vi "read_Mazak.vi"(8 "error in":errorcluster, 10 "Boolean":bool=TRUE, 11 "URL":string) -> (0 "machine":T2, 1 "c2":T4, 2 "c":T5, 3 "vr":T3, 4 "position":T1, 5 "br":T6, 7 "error out":errorcluster)   [LabVIEW 2014]
uses:
  <vilib>/addons/internet/NI_InternetTK_Core_VIs.lvlib
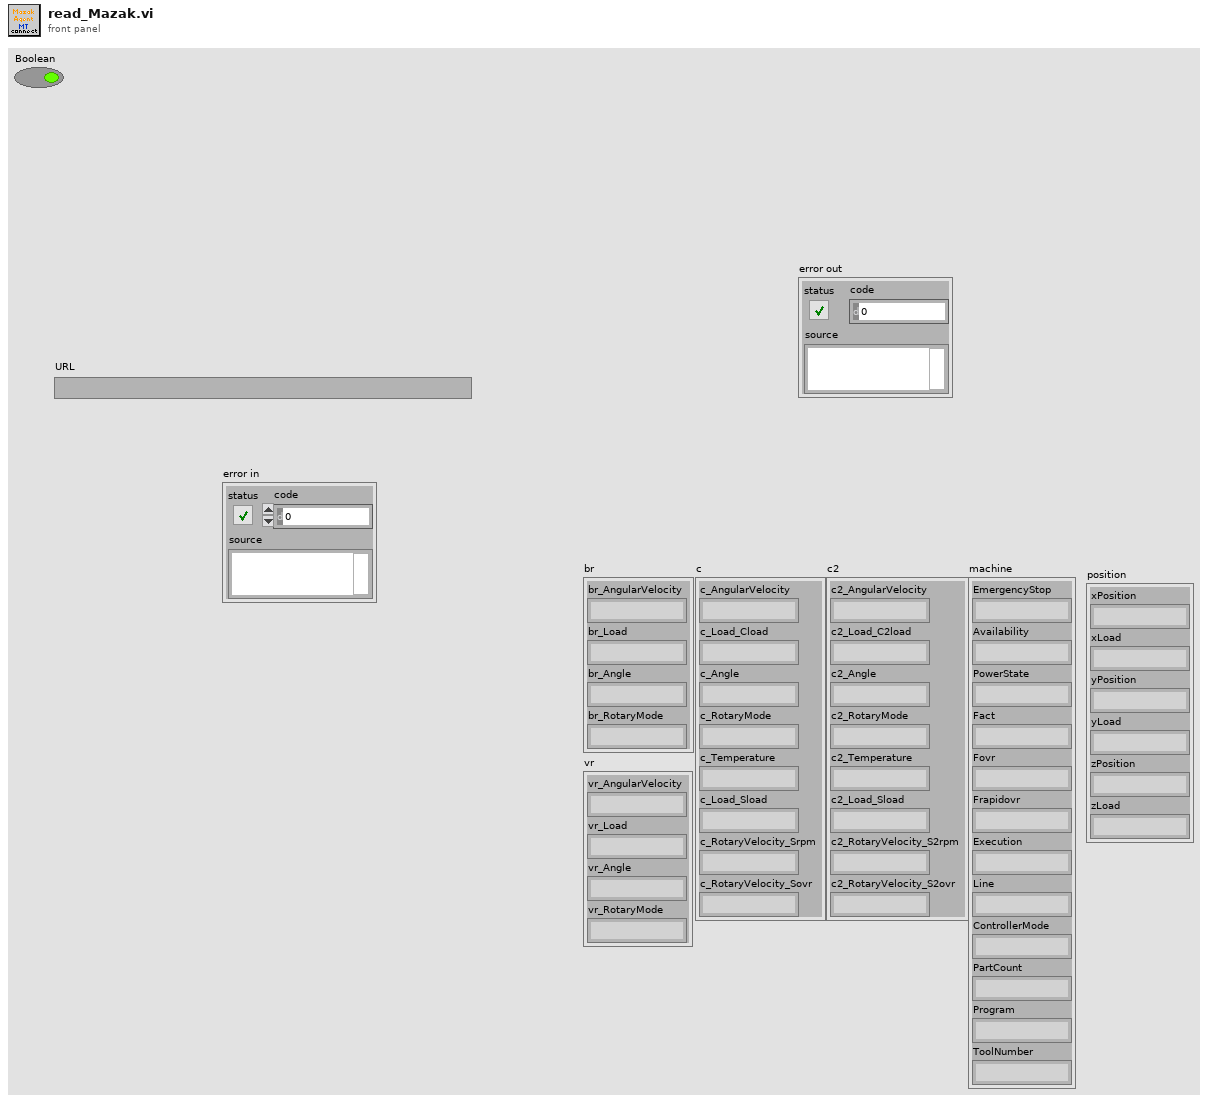
[diagram p1: front panel]
types:
  T1 = cluster{"xPosition":string, "xLoad":string, "yPosition":string, "yLoad":string, "zPosition":string, "zLoad":string}
  T2 = cluster{"EmergencyStop":string, "Availability":string, "PowerState":string, "Fact":string, "Fovr":string, "Frapidovr":string, "Execution":string, "Line":string, "ControllerMode":string, "PartCount":string, "Program":string, "ToolNumber":string}
  T3 = cluster{"vr_AngularVelocity":string, "vr_Load":string, "vr_Angle":string, "vr_RotaryMode":string}
  T4 = cluster{"c2_AngularVelocity":string, "c2_Load_C2load":string, "c2_Angle":string, "c2_RotaryMode":string, "c2_Temperature":string, "c2_Load_Sload":string, "c2_RotaryVelocity_S2rpm":string, "c2_RotaryVelocity_S2ovr":string}
  T5 = cluster{"c_AngularVelocity":string, "c_Load_Cload":string, "c_Angle":string, "c_RotaryMode":string, "c_Temperature":string, "c_Load_Sload":string, "c_RotaryVelocity_Srpm":string, "c_RotaryVelocity_Sovr":string}
  T6 = cluster{"br_AngularVelocity":string, "br_Load":string, "br_Angle":string, "br_RotaryMode":string}
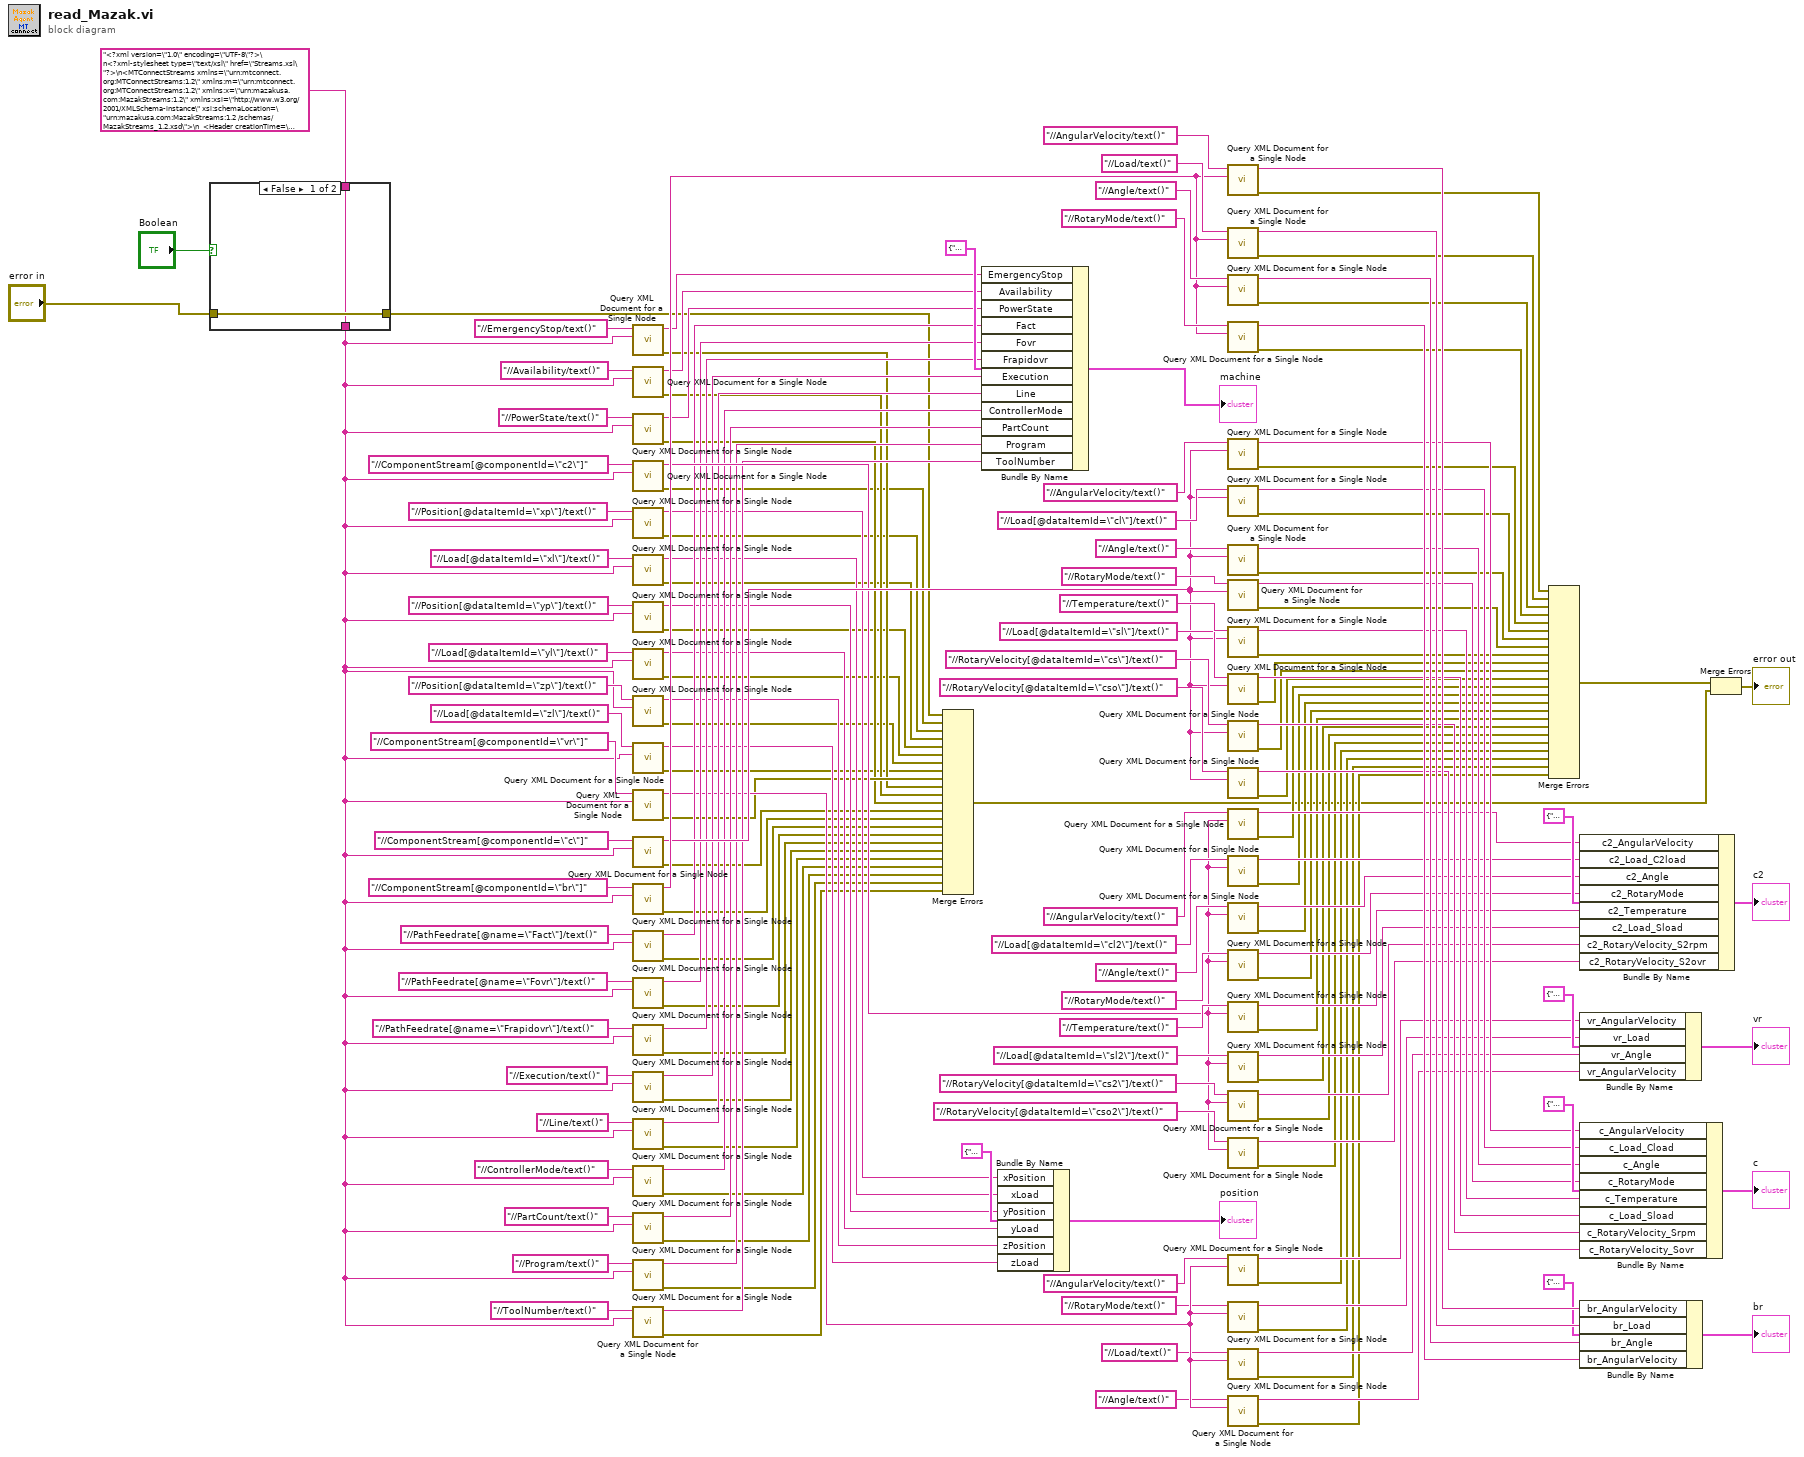
[diagram p0: block diagram]
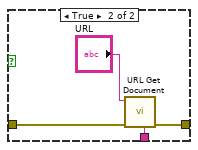
[diagram p2: hidden frame]
diagram:
  n1 = case shown="False" "Boolean" {
    tunnel: "error in" -> [w160 w164]
    tunnel: [w159 w163] -> w53
    tunnel: [w160 w161] -> w3
    tunnel: "<?xml version=\"1.0\" encoding=\"UTF-8\"?>\n<?xml-stylesheet type=\"text/xsl\" href=\"Streams.xsl\"?>\n<MTConnectStreams xmlns=\"urn:mtconnect.org:MTConnectStreams:1.2\" xmlns:m=\"urn:mtconnect.org:MTConnectStreams:1.2\" xmlns:x=\"urn:mazakusa.com:MazakStreams:1.2\" xmlns:xsi=\"http://www.w3.org/2001/XMLSchema-instance\" xsi:schemaLocation=\"urn:mazakusa.com:MazakStreams:1.2 /schemas/MazakStreams_1.2.xsd\">\n  <Header creationTime=\"2016-04-06T16:39:26Z\" sender=\"MAZATROL-PC\" instanceId=\"1459800093\" version=\"1.2.0.22\" bufferSize=\"16384\" nextSequence=\"535780\" firstSequence=\"519396\" lastSequence=\"535779\" />\n  <Streams>\n    <DeviceStream name=\"e-Series\" uuid=\"MAZAK-M7303290458\">\n      <ComponentStream component=\"Axes\" name=\"base\" componentId=\"a\">\n        <Condition>\n          <Normal dataItemId=\"servo\" timestamp=\"2016-04-04T20:01:46.125Z\" name=\"servo_cond\" sequence=\"82\" type=\"ACTUATOR\" />\n        </Condition>\n      </ComponentStream>\n      <ComponentStream component=\"Rotary\" name=\"B\" componentId=\"br\">\n        <Samples>\n          <AngularVelocity dataItemId=\"bf\" timestamp=\"2016-04-06T11:27:44.709Z\" name=\"Bfrt\" sequence=\"516876\">0</AngularVelocity>\n          <Load dataItemId=\"bl\" timestamp=\"2016-04-06T11:27:44.709Z\" name=\"Bload\" sequence=\"516877\">0</Load>\n          <Angle dataItemId=\"bpos\" timestamp=\"2016-04-06T11:27:44.709Z\" name=\"Bdeg\" sequence=\"516875\" subType=\"ACTUAL\">0</Angle>\n        </Samples>\n        <Events>\n          <RotaryMode dataItemId=\"brf\" timestamp=\"2016-04-04T20:01:33.224Z\" name=\"brfunc\" sequence=\"6\">UNAVAILABLE</RotaryMode>\n        </Events>\n        <Condition>\n          <Normal dataItemId=\"bt\" timestamp=\"2016-04-04T20:03:10.465Z\" name=\"Btravel\" sequence=\"97\" type=\"ANGLE\" />\n        </Condition>\n      </ComponentStream>\n      <ComponentStream component=\"Rotary\" name=\"C\" componentId=\"c\">\n        <Samples>\n          <AngularVelocity dataItemId=\"cf\" timestamp=\"2016-04-06T11:58:20.995Z\" name=\"Cfrt\" sequence=\"521223\">0</AngularVelocity>\n          <Load dataItemId=\"cl\" timestamp=\"2016-04-06T11:58:20.995Z\" name=\"Cload\" sequence=\"521224\">0</Load>\n          <Angle dataItemId=\"cpos\" timestamp=\"2016-04-06T11:58:20.995Z\" name=\"Cdeg\" sequence=\"521222\" subType=\"ACTUAL\">138.3637</Angle>\n          <RotaryVelocity dataItemId=\"cs\" timestamp=\"2016-04-06T11:39:30.023Z\" name=\"Srpm\" sequence=\"520012\" subType=\"ACTUAL\">0</RotaryVelocity>\n          <RotaryVelocity dataItemId=\"cso\" timestamp=\"2016-04-06T11:03:57.000Z\" name=\"Sovr\" sequence=\"509281\" subType=\"OVERRIDE\">100</RotaryVelocity>\n          <Temperature dataItemId=\"ctemp\" timestamp=\"2016-04-06T16:19:20.460Z\" name=\"Stemp\" sequence=\"534875\">23</Temperature>\n          <Load dataItemId=\"sl\" timestamp=\"2016-04-06T11:24:51.813Z\" name=\"Sload\" sequence=\"516066\">0</Load>\n        </Samples>\n        <Events>\n          <RotaryMode dataItemId=\"rf\" timestamp=\"2016-04-04T20:01:33.224Z\" name=\"crfunc\" sequence=\"46\">UNAVAILABLE</RotaryMode>\n        </Events>\n        <Condition>\n          <Normal dataItemId=\"ct\" timestamp=\"2016-04-04T20:03:10.465Z\" name=\"Ctravel\" sequence=\"98\" type=\"ANGLE\" />\n          <Normal dataItemId=\"spc\" timestamp=\"2016-04-04T20:03:10.465Z\" name=\"Sload_cond\" sequence=\"100\" type=\"LOAD\" />\n          <Normal dataItemId=\"tmp\" timestamp=\"2016-04-04T20:03:10.465Z\" name=\"Stemp_cond\" sequence=\"101\" type=\"TEMPERATURE\" />\n        </Condition>\n      </ComponentStream>\n      <ComponentStream component=\"Rotary\" name=\"C2\" componentId=\"c2\">\n        <Samples>\n          <AngularVelocity dataItemId=\"cf2\" timestamp=\"2016-04-04T20:01:33.224Z\" name=\"C2frt\" sequence=\"10\">UNAVAILABLE</AngularVelocity>\n          <Load dataItemId=\"cl2\" timestamp=\"2016-04-04T20:01:33.224Z\" name=\"C2load\" sequence=\"12\">UNAVAILABLE</Load>\n          <Angle dataItemId=\"cpos2\" timestamp=\"2016-04-04T20:01:33.224Z\" name=\"C2deg\" sequence=\"17\" subType=\"ACTUAL\">UNAVAILABLE</Angle>\n          <RotaryVelocity dataItemId=\"cs2\" timestamp=\"2016-04-04T20:01:33.224Z\" name=\"S2rpm\" sequence=\"19\" subType=\"ACTUAL\">UNAVAILABLE</RotaryVelocity>\n          <RotaryVelocity dataItemId=\"cso2\" timestamp=\"2016-04-04T20:01:33.224Z\" name=\"S2ovr\" sequence=\"21\" subType=\"OVERRIDE\">UNAVAILABLE</RotaryVelocity>\n          <Temperature dataItemId=\"ctemp2\" timestamp=\"2016-04-04T20:01:33.224Z\" name=\"S2temp\" sequence=\"25\">UNAVAILABLE</Temperature>\n          <Load dataItemId=\"sl2\" timestamp=\"2016-04-04T20:01:33.224Z\" name=\"S2load\" sequence=\"51\">UNAVAILABLE</Load>\n        </Samples>\n        <Events>\n          <RotaryMode dataItemId=\"rf2\" timestamp=\"2016-04-04T20:01:33.224Z\" name=\"c2rfunc\" sequence=\"47\">UNAVAILABLE</RotaryMode>\n        </Events>\n        <Condition>\n          <Unavailable dataItemId=\"ct2\" timestamp=\"2016-04-04T20:01:33.224Z\" name=\"C2travel\" sequence=\"23\" type=\"ANGLE\" />\n          <Unavailable dataItemId=\"spc2\" timestamp=\"2016-04-04T20:01:33.224Z\" name=\"S2load_cond\" sequence=\"53\" type=\"LOAD\" />\n          <Unavailable dataItemId=\"tmp2\" timestamp=\"2016-04-04T20:01:33.224Z\" name=\"S2temp_cond\" sequence=\"60\" type=\"TEMPERATURE\" />\n        </Condition>\n      </ComponentStream>\n      <ComponentStream component=\"Controller\" name=\"controller\" componentId=\"cont\">\n        <Events>\n          <EmergencyStop dataItemId=\"estop\" timestamp=\"2016-04-05T13:35:23.466Z\" name=\"estop\" sequence=\"199888\">ARMED</EmergencyStop>\n        </Events>\n        <Condition>\n          <Normal dataItemId=\"ccond\" timestamp=\"2016-04-04T20:01:46.125Z\" name=\"comms_cond\" sequence=\"83\" type=\"COMMUNICATIONS\" />\n          <Normal dataItemId=\"logic\" timestamp=\"2016-04-06T16:39:04.533Z\" name=\"logic_cond\" sequence=\"535758\" type=\"LOGIC_PROGRAM\" />\n          <Normal dataItemId=\"system\" timestamp=\"2016-04-06T11:27:43.618Z\" name=\"system_cond\" sequence=\"516862\" type=\"SYSTEM\" />\n        </Condition>\n      </ComponentStream>\n      <ComponentStream component=\"Coolant\" name=\"coolant\" componentId=\"coolant\">\n        <Condition>\n          <Normal dataItemId=\"coollevel\" timestamp=\"2016-04-06T08:34:22.682Z\" name=\"coolant_level\" sequence=\"435644\" type=\"LEVEL\" />\n          <Normal dataItemId=\"coolpress\" timestamp=\"2016-04-04T20:01:46.125Z\" name=\"coolant_pres\" sequence=\"90\" type=\"PRESSURE\" />\n          <Normal dataItemId=\"cooltemp\" timestamp=\"2016-04-04T20:01:46.125Z\" name=\"coolant_temp\" sequence=\"89\" type=\"TEMPERATURE\" />\n        </Condition>\n      </ComponentStream>\n      <ComponentStream component=\"Device\" name=\"e-Series\" componentId=\"d1\">\n        <Events>\n          <Availability dataItemId=\"avail\" timestamp=\"2016-04-04T20:01:46.125Z\" sequence=\"81\">AVAILABLE</Availability>\n          <AssetChanged dataItemId=\"d1_asset_chg\" timestamp=\"2016-04-04T20:01:33.224Z\" sequence=\"27\" assetType=\"\">UNAVAILABLE</AssetChanged>\n        </Events>\n      </ComponentStream>\n      <ComponentStream component=\"Electric\" name=\"electric\" componentId=\"elec\">\n        <Events>\n          <PowerState dataItemId=\"pwr\" timestamp=\"2016-04-04T20:03:10.465Z\" name=\"power\" sequence=\"93\">ON</PowerState>\n        </Events>\n        <Condition>\n          <Normal dataItemId=\"pwrt\" timestamp=\"2016-04-04T20:01:46.125Z\" name=\"electric_temp\" sequence=\"92\" type=\"TEMPERATURE\" />\n        </Condition>\n      </ComponentStream>\n      <ComponentStream component=\"Hydraulic\" name=\"hydraulic\" componentId=\"hydraulic\">\n        <Condition>\n          <Normal dataItemId=\"hyd\" timestamp=\"2016-04-04T20:01:46.125Z\" name=\"hydra_cond\" sequence=\"87\" type=\"PRESSURE\" />\n        </Condition>\n      </ComponentStream>\n      <ComponentStream component=\"Path\" name=\"path\" componentId=\"path1\">\n        <Samples>\n          <AccumulatedTime dataItemId=\"atime\" timestamp=\"2016-04-06T11:39:37.593Z\" name=\"auto_time\" sequence=\"520070\" subType=\"x:AUTO\">32773294</AccumulatedTime>\n          <AccumulatedTime dataItemId=\"ctime\" timestamp=\"2016-04-06T11:39:28.947Z\" name=\"cut_time\" sequence=\"520008\" subType=\"x:CUT\">14501503</AccumulatedTime>\n          <PathFeedrate dataItemId=\"pf\" timestamp=\"2016-04-06T11:58:20.995Z\" name=\"Fact\" sequence=\"521225\" subType=\"ACTUAL\">0</PathFeedrate>\n          <PathFeedrate dataItemId=\"pfo\" timestamp=\"2016-04-06T11:24:53.997Z\" name=\"Fovr\" sequence=\"516086\" subType=\"OVERRIDE\">100</PathFeedrate>\n          <PathFeedrate dataItemId=\"pfr\" timestamp=\"2016-04-06T11:39:40.145Z\" name=\"Frapidovr\" sequence=\"520075\" subType=\"OVERRIDE\">100</PathFeedrate>\n          <AccumulatedTime dataItemId=\"yltime\" timestamp=\"2016-04-06T16:39:26.264Z\" name=\"total_time\" sequence=\"535779\" subType=\"x:TOTAL\">71278506</AccumulatedTime>\n        </Samples>\n        <Events>\n          <Execution dataItemId=\"exec\" timestamp=\"2016-04-06T11:39:40.145Z\" name=\"execution\" sequence=\"520074\">STOPPED</Execution>\n          <Line dataItemId=\"ln\" timestamp=\"2016-04-06T11:39:37.593Z\" name=\"line\" sequence=\"520067\">0</Line>\n          <ControllerMode dataItemId=\"mode\" timestamp=\"2016-04-06T11:39:40.145Z\" name=\"mode\" sequence=\"520076\">MANUAL</ControllerMode>\n          <PartCount dataItemId=\"pc\" timestamp=\"2016-04-04T20:03:11.916Z\" name=\"PartCountAct\" sequence=\"139\">0</PartCount>\n          <x:ProgramComment dataItemId=\"pcmt\" timestamp=\"2016-04-05T19:02:24.670Z\" name=\"program_cmt\" sequence=\"265033\" />\n          <Program dataItemId=\"pgm\" timestamp=\"2016-04-06T08:34:29.153Z\" name=\"program\" sequence=\"435652\">555885</Program>\n          <x:PalletNum dataItemId=\"pltnum\" timestamp=\"2016-04-04T20:03:13.211Z\" name=\"pallet_num\" sequence=\"143\">2</x:PalletNum>\n          <x:SequenceNumber dataItemId=\"seq\" timestamp=\"2016-04-06T11:39:37.593Z\" name=\"sequenceNum\" sequence=\"520069\">0</x:SequenceNumber>\n          <x:ProgramComment dataItemId=\"spcmt\" timestamp=\"2016-04-06T08:28:01.332Z\" name=\"subprogram_cmt\" sequence=\"434132\" subType=\"x:SUB\" />\n          <Program dataItemId=\"spgm\" timestamp=\"2016-04-06T11:27:35.278Z\" name=\"subprogram\" sequence=\"516799\" subType=\"x:SUB\" />\n          <ToolNumber dataItemId=\"tid\" timestamp=\"2016-04-06T11:27:29.889Z\" name=\"Tool_number\" sequence=\"516764\">16</ToolNumber>\n          <x:ToolGroup dataItemId=\"tid1\" timestamp=\"2016-04-04T20:03:11.916Z\" name=\"Tool_group\" sequence=\"136\">0</x:ToolGroup>\n          <x:ToolSuffix dataItemId=\"tsuf1\" timestamp=\"2016-04-04T20:01:33.224Z\" name=\"Tool_suffix\" sequence=\"61\">UNAVAILABLE</x:ToolSuffix>\n          <x:Unit dataItemId=\"unit\" timestamp=\"2016-04-04T20:03:11.916Z\" name=\"unitNum\" sequence=\"138\">0</x:Unit>\n        </Events>\n        <Condition>\n          <Normal dataItemId=\"motion\" timestamp=\"2016-04-05T15:21:48.586Z\" name=\"motion_cond\" sequence=\"233870\" type=\"MOTION_PROGRAM\" />\n          <Normal dataItemId=\"path_system\" timestamp=\"2016-04-04T20:03:10.465Z\" name=\"path_system\" sequence=\"103\" type=\"SYSTEM\" />\n        </Condition>\n      </ComponentStream>\n      <ComponentStream component=\"Pneumatic\" name=\"pneumatic\" componentId=\"pneumatic\">\n        <Condition>\n          <Normal dataItemId=\"pneupress\" timestamp=\"2016-04-05T08:03:22.286Z\" name=\"pneu_cond\" sequence=\"131871\" type=\"PRESSURE\" />\n        </Condition>\n      </ComponentStream>\n      <ComponentStream component=\"Rotary\" name=\"V\" componentId=\"vr\">\n        <Samples>\n          <AngularVelocity dataItemId=\"vf\" timestamp=\"2016-04-04T20:03:11.916Z\" name=\"Vfrt\" sequence=\"122\">0</AngularVelocity>\n          <Load dataItemId=\"vl\" timestamp=\"2016-04-04T20:03:11.916Z\" name=\"Vload\" sequence=\"123\">0</Load>\n          <Angle dataItemId=\"vpos\" timestamp=\"2016-04-04T20:03:11.916Z\" name=\"Vdeg\" sequence=\"121\" subType=\"ACTUAL\">0</Angle>\n        </Samples>\n        <Events>\n          <RotaryMode dataItemId=\"vrf\" timestamp=\"2016-04-04T20:01:33.224Z\" name=\"vrfunc\" sequence=\"66\">UNAVAILABLE</RotaryMode>\n        </Events>\n        <Condition>\n          <Normal dataItemId=\"vt\" timestamp=\"2016-04-04T20:03:10.465Z\" name=\"Vtravel\" sequence=\"99\" type=\"ANGLE\" />\n        </Condition>\n      </ComponentStream>\n      <ComponentStream component=\"Linear\" name=\"X\" componentId=\"x\">\n        <Samples>\n          <AxisFeedrate dataItemId=\"xf\" timestamp=\"2016-04-06T11:58:12.291Z\" name=\"Xfrt\" sequence=\"521195\">0</AxisFeedrate>\n          <Load dataItemId=\"xl\" timestamp=\"2016-04-06T15:27:46.990Z\" name=\"Xload\" sequence=\"532523\">2</Load>\n          <Position dataItemId=\"xp\" timestamp=\"2016-04-06T11:58:11.214Z\" name=\"Xabs\" sequence=\"521190\" subType=\"ACTUAL\">1334.898524</Position>\n        </Samples>\n        <Condition>\n          <Normal dataItemId=\"xt\" timestamp=\"2016-04-05T04:05:33.224Z\" name=\"Xtravel\" sequence=\"102549\" type=\"POSITION\" />\n        </Condition>\n      </ComponentStream>\n      <ComponentStream component=\"Linear\" name=\"Y\" componentId=\"y\">\n        <Samples>\n          <AxisFeedrate dataItemId=\"yf\" timestamp=\"2016-04-06T11:39:34.344Z\" name=\"Yfrt\" sequence=\"520050\">0</AxisFeedrate>\n          <Load dataItemId=\"yl\" timestamp=\"2016-04-06T11:39:34.344Z\" name=\"Yload\" sequence=\"520051\">3</Load>\n          <Position dataItemId=\"yp\" timestamp=\"2016-04-06T11:39:34.344Z\" name=\"Yabs\" sequence=\"520049\" subType=\"ACTUAL\">529.98243</Position>\n        </Samples>\n        <Condition>\n          <Normal dataItemId=\"yt\" timestamp=\"2016-04-04T20:03:10.465Z\" name=\"Ytravel\" sequence=\"95\" type=\"POSITION\" />\n        </Condition>\n      </ComponentStream>\n      <ComponentStream component=\"Linear\" name=\"Z\" componentId=\"z\">\n        <Samples>\n          <AxisFeedrate dataItemId=\"zf\" timestamp=\"2016-04-06T11:39:32.176Z\" name=\"Zfrt\" sequence=\"520031\">0</AxisFeedrate>\n          <Load dataItemId=\"zl\" timestamp=\"2016-04-06T11:39:33.268Z\" name=\"Zload\" sequence=\"520044\">42</Load>\n          <Position dataItemId=\"zp\" timestamp=\"2016-04-06T11:39:40.145Z\" name=\"Zabs\" sequence=\"520073\" subType=\"ACTUAL\">936.407957</Position>\n        </Samples>\n        <Condition>\n          <Normal dataItemId=\"zt\" timestamp=\"2016-04-04T20:03:10.465Z\" name=\"Ztravel\" sequence=\"96\" type=\"POSITION\" />\n        </Condition>\n      </ComponentStream>\n    </DeviceStream>\n  </Streams>\n</MTConnectStreams>\n" ("XML Input") -> [w159 _]
    frame False {
    }
    frame True {
      n2 = call <vilib>:"URL Get Document.vi"("error in (no error)"=w164, "URL"="URL") -> ("error out"=w161:errorcluster, "content"=w163:string)  [unwired: 5 in, 3 out]
    }
  }
  n3 = call "Query XML Document for a Single Node.vi"("XML document"=w53, "XPath expression"="//EmergencyStop/text()") -> ("error out"=w27:errorcluster, "Result XML"=w96:string)  [unwired: 7 in, 1 out]
  n4 = call "Query XML Document for a Single Node.vi"("XML document"=w53, "XPath expression"="//Availability/text()") -> ("error out"=w26:errorcluster, "Result XML"=w95:string)  [unwired: 7 in, 1 out]
  n5 = call "Query XML Document for a Single Node.vi"("XML document"=w53, "XPath expression"="//PowerState/text()") -> ("error out"=w25:errorcluster, "Result XML"=w94:string)  [unwired: 7 in, 1 out]
  n6 = call "Query XML Document for a Single Node.vi"("XML document"=w53, "XPath expression"="//ComponentStream[@componentId=\"c2\"]") -> ("error out"=w7:errorcluster, "Result XML"=w134:string)  [unwired: 7 in, 1 out]
  n7 = call "Query XML Document for a Single Node.vi"("XML document"=w53, "XPath expression"="//Position[@dataItemId=\"xp\"]/text()") -> ("error out"=w8:errorcluster, "Result XML"=w66:string)  [unwired: 7 in, 1 out]
  n8 = call "Query XML Document for a Single Node.vi"("XML document"=w53, "XPath expression"="//Load[@dataItemId=\"xl\"]/text()") -> ("error out"=w9:errorcluster, "Result XML"=w65:string)  [unwired: 7 in, 1 out]
  n9 = call "Query XML Document for a Single Node.vi"("XML document"=w53, "XPath expression"="//Position[@dataItemId=\"yp\"]/text()") -> ("error out"=w10:errorcluster, "Result XML"=w64:string)  [unwired: 7 in, 1 out]
  n10 = call "Query XML Document for a Single Node.vi"("XML document"=w53, "XPath expression"="//Load[@dataItemId=\"yl\"]/text()") -> ("error out"=w11:errorcluster, "Result XML"=w63:string)  [unwired: 7 in, 1 out]
  n11 = call "Query XML Document for a Single Node.vi"("XML document"=w53, "XPath expression"="//Position[@dataItemId=\"zp\"]/text()") -> ("error out"=w12:errorcluster, "Result XML"=w62:string)  [unwired: 7 in, 1 out]
  n12 = call "Query XML Document for a Single Node.vi"("XML document"=w53, "XPath expression"="//Load[@dataItemId=\"zl\"]/text()") -> ("error out"=w13:errorcluster, "Result XML"=w61:string)  [unwired: 7 in, 1 out]
  n13 = call "Query XML Document for a Single Node.vi"("XML document"=w53, "XPath expression"="//ComponentStream[@componentId=\"vr\"]") -> ("error out"=w28:errorcluster, "Result XML"=w84:string)  [unwired: 7 in, 1 out]
  n14 = call "Query XML Document for a Single Node.vi"("XML document"=w53, "XPath expression"="//ComponentStream[@componentId=\"c\"]") -> ("error out"=w21:errorcluster, "Result XML"=w143:string)  [unwired: 7 in, 1 out]
  n15 = call "Query XML Document for a Single Node.vi"("XML document"=w53, "XPath expression"="//ComponentStream[@componentId=\"br\"]") -> ("error out"=w20:errorcluster, "Result XML"=w149:string)  [unwired: 7 in, 1 out]
  n16 = call "Query XML Document for a Single Node.vi"("XML document"=w53, "XPath expression"="//PathFeedrate[@name=\"Fact\"]/text()") -> ("error out"=w24:errorcluster, "Result XML"=w93:string)  [unwired: 7 in, 1 out]
  n17 = call "Query XML Document for a Single Node.vi"("XML document"=w53, "XPath expression"="//PathFeedrate[@name=\"Fovr\"]/text()") -> ("error out"=w23:errorcluster, "Result XML"=w92:string)  [unwired: 7 in, 1 out]
  n18 = call "Query XML Document for a Single Node.vi"("XML document"=w53, "XPath expression"="//PathFeedrate[@name=\"Frapidovr\"]/text()") -> ("error out"=w22:errorcluster, "Result XML"=w91:string)  [unwired: 7 in, 1 out]
  n19 = call "Query XML Document for a Single Node.vi"("XML document"=w53, "XPath expression"="//Execution/text()") -> ("error out"=w19:errorcluster, "Result XML"=w90:string)  [unwired: 7 in, 1 out]
  n20 = call "Query XML Document for a Single Node.vi"("XML document"=w53, "XPath expression"="//Line/text()") -> ("error out"=w18:errorcluster, "Result XML"=w89:string)  [unwired: 7 in, 1 out]
  n21 = call "Query XML Document for a Single Node.vi"("XML document"=w53, "XPath expression"="//ControllerMode/text()") -> ("error out"=w17:errorcluster, "Result XML"=w88:string)  [unwired: 7 in, 1 out]
  n22 = call "Query XML Document for a Single Node.vi"("XML document"=w53, "XPath expression"="//PartCount/text()") -> ("error out"=w16:errorcluster, "Result XML"=w87:string)  [unwired: 7 in, 1 out]
  n23 = call "Query XML Document for a Single Node.vi"("XML document"=w53, "XPath expression"="//Program/text()") -> ("error out"=w15:errorcluster, "Result XML"=w86:string)  [unwired: 7 in, 1 out]
  n24 = call "Query XML Document for a Single Node.vi"("XML document"=w53, "XPath expression"="//ToolNumber/text()") -> ("error out"=w14:errorcluster, "Result XML"=w85:string)  [unwired: 7 in, 1 out]
  n25 = Merge Errors(w3, w7, w8, w9, w10, w11, w12, w13, w28, w27, w26, w25, w21, w20, w24, w23, w22, w19, w18, w17, w16, w15, w14) -> (w5:errorcluster)
  n26 = Bundle By Name(cluster=T2 {"EmergencyStop"="ARMED", "Availability"="AVAILABLE", "PowerState"="ON", "Fact"="0", "Fovr"="100", "Frapidovr"="100", "Execution"="STOPPED", "Line"="0", "ControllerMode"="MANUAL", "PartCount"="0", "Program"="0", "ToolNumber"="0"} ("input cluster"), "EmergencyStop"=w96, "Availability"=w95, "PowerState"=w94, "Fact"=w93, "Fovr"=w92, "Frapidovr"=w91, "Execution"=w90, "Line"=w89, "ControllerMode"=w88, "PartCount"=w87, "Program"=w86, "ToolNumber"=w85) -> (→"machine":T2)
  n27 = Bundle By Name(cluster=T1 {"xPosition"="", "xLoad"="", "yPosition"="", "yLoad"="", "zPosition"="", "zLoad"=""} ("input cluster"), "xPosition"=w66, "xLoad"=w65, "yPosition"=w64, "yLoad"=w63, "zPosition"=w62, "zLoad"=w61) -> (→"position":T1)
  n28 = call "Query XML Document for a Single Node.vi"("XML document"=w149, "XPath expression"="//AngularVelocity/text()") -> ("error out"=w52:errorcluster, "Result XML"=w133:string)  [unwired: 7 in, 1 out]
  n29 = call "Query XML Document for a Single Node.vi"("XML document"=w149, "XPath expression"="//Load/text()") -> ("error out"=w51:errorcluster, "Result XML"=w132:string)  [unwired: 7 in, 1 out]
  n30 = call "Query XML Document for a Single Node.vi"("XML document"=w149, "XPath expression"="//Angle/text()") -> ("error out"=w50:errorcluster, "Result XML"=w131:string)  [unwired: 7 in, 1 out]
  n31 = call "Query XML Document for a Single Node.vi"("XML document"=w149, "XPath expression"="//RotaryMode/text()") -> ("error out"=w49:errorcluster, "Result XML"=w130:string)  [unwired: 7 in, 1 out]
  n32 = call "Query XML Document for a Single Node.vi"("XML document"=w143, "XPath expression"="//AngularVelocity/text()") -> ("error out"=w48:errorcluster, "Result XML"=w127:string)  [unwired: 7 in, 1 out]
  n33 = call "Query XML Document for a Single Node.vi"("XML document"=w143, "XPath expression"="//Load[@dataItemId=\"cl\"]/text()") -> ("error out"=w47:errorcluster, "Result XML"=w126:string)  [unwired: 7 in, 1 out]
  n34 = call "Query XML Document for a Single Node.vi"("XML document"=w143, "XPath expression"="//Angle/text()") -> ("error out"=w46:errorcluster, "Result XML"=w125:string)  [unwired: 7 in, 1 out]
  n35 = call "Query XML Document for a Single Node.vi"("XML document"=w143, "XPath expression"="//RotaryMode/text()") -> ("error out"=w45:errorcluster, "Result XML"=w124:string)  [unwired: 7 in, 1 out]
  n36 = call "Query XML Document for a Single Node.vi"("XML document"=w143, "XPath expression"="//Temperature/text()") -> ("error out"=w44:errorcluster, "Result XML"=w123:string)  [unwired: 7 in, 1 out]
  n37 = call "Query XML Document for a Single Node.vi"("XML document"=w143, "XPath expression"="//Load[@dataItemId=\"sl\"]/text()") -> ("error out"=w43:errorcluster, "Result XML"=w122:string)  [unwired: 7 in, 1 out]
  n38 = call "Query XML Document for a Single Node.vi"("XML document"=w143, "XPath expression"="//RotaryVelocity[@dataItemId=\"cs\"]/text()") -> ("error out"=w42:errorcluster, "Result XML"=w121:string)  [unwired: 7 in, 1 out]
  n39 = call "Query XML Document for a Single Node.vi"("XML document"=w143, "XPath expression"="//RotaryVelocity[@dataItemId=\"cso\"]/text()") -> ("error out"=w41:errorcluster, "Result XML"=w120:string)  [unwired: 7 in, 1 out]
  n40 = call "Query XML Document for a Single Node.vi"("XML document"=w134, "XPath expression"="//AngularVelocity/text()") -> ("error out"=w40:errorcluster, "Result XML"=w118:string)  [unwired: 7 in, 1 out]
  n41 = call "Query XML Document for a Single Node.vi"("XML document"=w134, "XPath expression"="//Load[@dataItemId=\"cl2\"]/text()") -> ("error out"=w39:errorcluster, "Result XML"=w117:string)  [unwired: 7 in, 1 out]
  n42 = call "Query XML Document for a Single Node.vi"("XML document"=w134, "XPath expression"="//Angle/text()") -> ("error out"=w38:errorcluster, "Result XML"=w116:string)  [unwired: 7 in, 1 out]
  n43 = call "Query XML Document for a Single Node.vi"("XML document"=w134, "XPath expression"="//RotaryMode/text()") -> ("error out"=w37:errorcluster, "Result XML"=w115:string)  [unwired: 7 in, 1 out]
  n44 = call "Query XML Document for a Single Node.vi"("XML document"=w134, "XPath expression"="//Temperature/text()") -> ("error out"=w36:errorcluster, "Result XML"=w114:string)  [unwired: 7 in, 1 out]
  n45 = call "Query XML Document for a Single Node.vi"("XML document"=w134, "XPath expression"="//Load[@dataItemId=\"sl2\"]/text()") -> ("error out"=w35:errorcluster, "Result XML"=w113:string)  [unwired: 7 in, 1 out]
  n46 = call "Query XML Document for a Single Node.vi"("XML document"=w134, "XPath expression"="//RotaryVelocity[@dataItemId=\"cs2\"]/text()") -> ("error out"=w34:errorcluster, "Result XML"=w112:string)  [unwired: 7 in, 1 out]
  n47 = call "Query XML Document for a Single Node.vi"("XML document"=w134, "XPath expression"="//RotaryVelocity[@dataItemId=\"cso2\"]/text()") -> ("error out"=w33:errorcluster, "Result XML"=w111:string)  [unwired: 7 in, 1 out]
  n48 = call "Query XML Document for a Single Node.vi"("XML document"=w84, "XPath expression"="//AngularVelocity/text()") -> ("error out"=w32:errorcluster, "Result XML"=w77:string)  [unwired: 7 in, 1 out]
  n49 = call "Query XML Document for a Single Node.vi"("XML document"=w84, "XPath expression"="//RotaryMode/text()") -> ("error out"=w31:errorcluster, "Result XML"=w76:string)  [unwired: 7 in, 1 out]
  n50 = call "Query XML Document for a Single Node.vi"("XML document"=w84, "XPath expression"="//Load/text()") -> ("error out"=w30:errorcluster, "Result XML"=w75:string)  [unwired: 7 in, 1 out]
  n51 = call "Query XML Document for a Single Node.vi"("XML document"=w84, "XPath expression"="//Angle/text()") -> ("error out"=w29:errorcluster, "Result XML"=w74:string)  [unwired: 7 in, 1 out]
  n52 = Merge Errors(w52, w51, w50, w49, w48, w47, w46, w45, w44, w43, w42, w41, w40, w39, w38, w37, w36, w35, w34, w33, w32, w31, w30, w29) -> (w6:errorcluster)
  n53 = Bundle By Name(cluster=T4 {"c2_AngularVelocity"="UNAVAILABLE", "c2_Load_C2load"="UNAVAILABLE", "c2_Angle"="UNAVAILABLE", "c2_RotaryMode"="UNAVAILABLE", "c2_Temperature"="UNAVAILABLE", "c2_Load_Sload"="UNAVAILABLE", "c2_RotaryVelocity_S2rpm"="UNAVAILABLE", "c2_RotaryVelocity_S2ovr"="UNAVAILABLE"} ("input cluster"), "c2_AngularVelocity"=w118, "c2_Load_C2load"=w117, "c2_Angle"=w116, "c2_RotaryMode"=w115, "c2_Temperature"=w114, "c2_Load_Sload"=w113, "c2_RotaryVelocity_S2rpm"=w112, "c2_RotaryVelocity_S2ovr"=w111) -> (→"c2":T4)
  n54 = Bundle By Name(cluster=T3 {"vr_AngularVelocity"="0", "vr_Load"="0", "vr_Angle"="0", "vr_RotaryMode"="UNAVAILABLE"} ("input cluster"), "vr_AngularVelocity"=w77, "vr_Load"=w76, "vr_Angle"=w75, "vr_AngularVelocity"=w74) -> (→"vr":T3)
  n55 = Bundle By Name(cluster=T5 {"c_AngularVelocity"="0", "c_Load_Cload"="0", "c_Angle"="138.3637", "c_RotaryMode"="UNAVAILABLE", "c_Temperature"="23", "c_Load_Sload"="0", "c_RotaryVelocity_Srpm"="0", "c_RotaryVelocity_Sovr"="100"} ("input cluster"), "c_AngularVelocity"=w127, "c_Load_Cload"=w126, "c_Angle"=w125, "c_RotaryMode"=w124, "c_Temperature"=w123, "c_Load_Sload"=w122, "c_RotaryVelocity_Srpm"=w121, "c_RotaryVelocity_Sovr"=w120) -> (→"c":T5)
  n56 = Bundle By Name(cluster=T6 {"br_AngularVelocity"="0", "br_Load"="0", "br_Angle"="0", "br_RotaryMode"="UNAVAILABLE"} ("input cluster"), "br_AngularVelocity"=w133, "br_Load"=w132, "br_Angle"=w131, "br_AngularVelocity"=w130) -> (→"br":T6)
  n57 = Merge Errors(w6, w5) -> (→"error out":errorcluster)
